vi "Práctica01_Ejercicio2_2.vi"() -> ()   [LabVIEW 2020]
uses:
  <vilib>/numeric/Random Number (Range) DBL.vi
panel:
  out "Waveform Chart":dbl[](graph)
  out "min value":dbl
  out "max value":dbl
  out "Datos organizados":dbl[][](array[numeric])
  out "Filtro EMA":dbl[](array[numeric])
  out "Fahrenheit":dbl[](array[numeric])
  out "Centigrados-Or":dbl[](array[numeric])
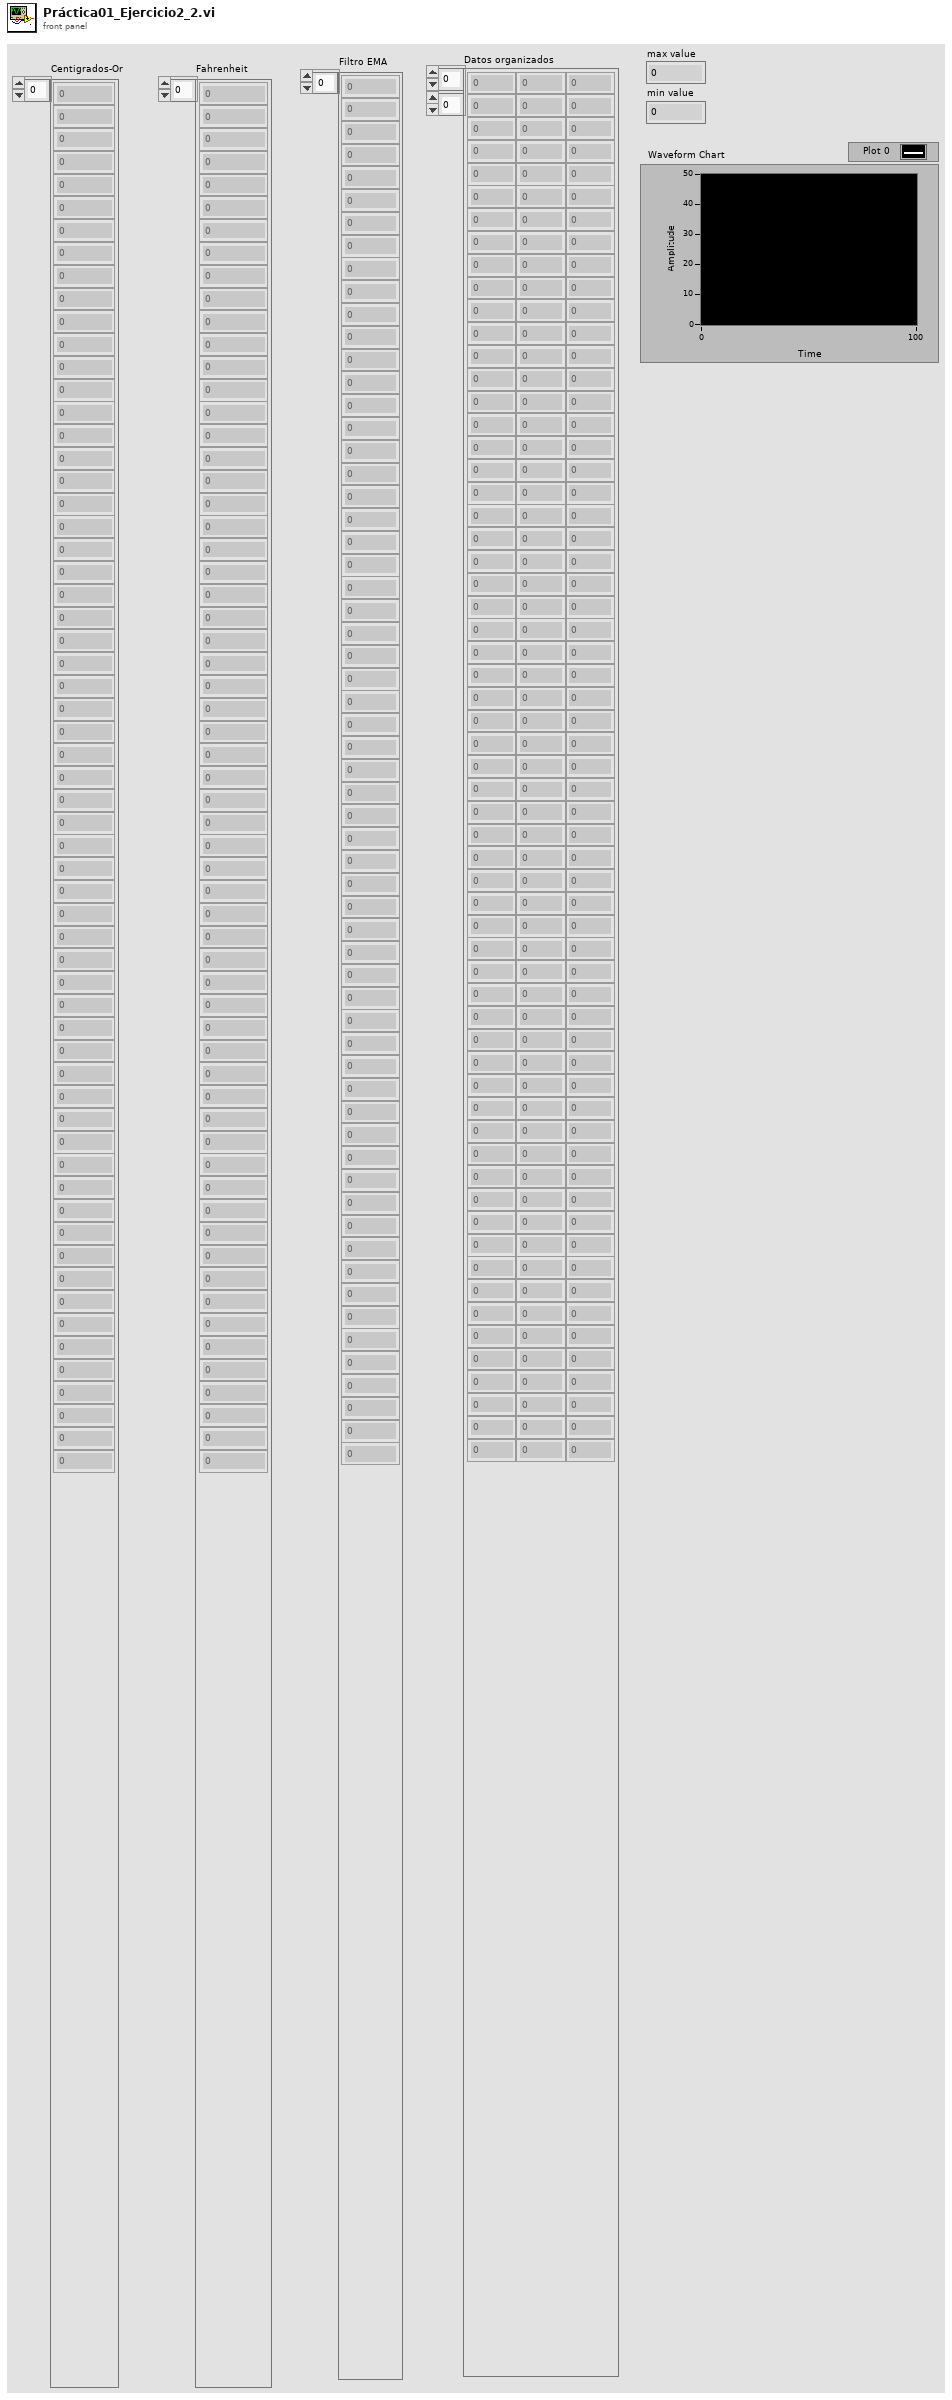
[diagram p1: front panel]
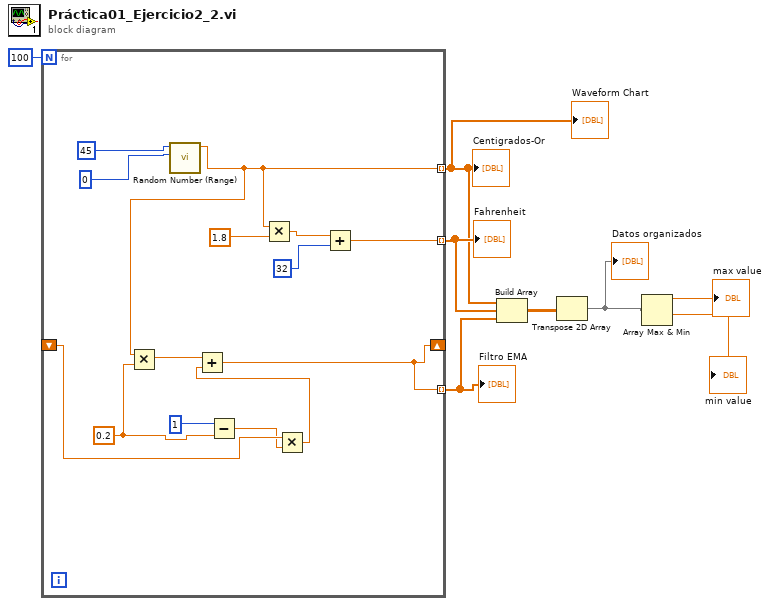
[diagram p0: block diagram]
diagram:
  n1 = for {
    N: 100 -> [_]
    tunnel: [w13] -> w1 mode=indexing
    tunnel: [w17] -> w7 mode=indexing
    shift-right: [w9] -> _
    shift-left: _ -> [w11]
    tunnel: [w9] -> w6 mode=indexing
    w14 = 0.2
    n2 = call-poly <vilib>:"Random Number (Range).vi"("lower bound (0)"=0, "upper bound (100)"=45) -> ("number"=w13:dbl)  [unwired: 9 in]
    n3 = Multiply(x=w13, y=w14) -> (x*y=w16:dbl)
    n4 = Subtract(x=1, y=w14) -> (x-y=w10:dbl)
    n5 = Multiply(x=w13, y=1.8) -> (x*y=w18:dbl)
    n6 = Multiply(x=w11, y=w10) -> (x*y=w12:dbl)
    n7 = Add(x=w16, y=w12) -> (x+y=w9:dbl)
    n8 = Add(x=w18, y=32) -> (x+y=w17:dbl)
  }
  "Centigrados-Or" <- w1
  "Fahrenheit" <- w7
  "Filtro EMA" <- w6
  "Waveform Chart" <- w1
  n9 = Build Array(w1, w7, w6) -> (w5:dbl[][])
  n10 = Transpose 2D Array(2D array=w5) -> (transposed array=w4:dbl[][])
  "Datos organizados" <- w4
  n11 = Array Max & Min(array=w4) -> (max value=→"max value":dbl, min value=→"min value":dbl)  [unwired: 2 out]
